vi "write_master_file.vi"(8 "error in (no error)":errorcluster, 10 "setup file paths":string, 11 "master file path":path) -> (0 "error out":errorcluster)   [LabVIEW 2017, in "worker.lvlib"]
uses:
  worker.lvlib
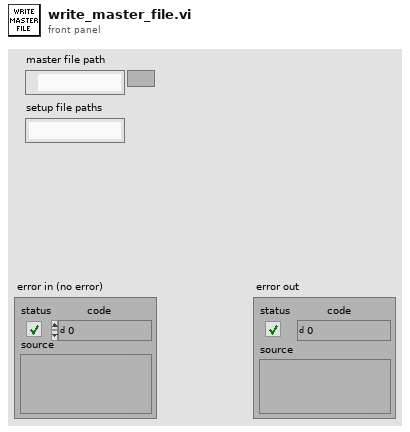
[diagram p1: front panel]
types:
  T1 = enum16{"open", "replace", "create", "open or create", "replace or create", "replace or create with confirmation"}
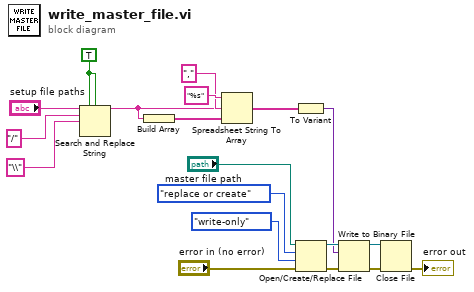
[diagram p0: block diagram]
diagram:
  w1 = TRUE ("replace all? (F)")
  n1 = Search and Replace String(replace all?=w1, case sensitive?=w1, input string="setup file paths", search string="/", replace string="\\" ("replace string (\"\")")) -> (result string=w4:string)  [unwired: 3 in, 3 out]
  n2 = Build Array(w4) -> (w8:string[])
  n3 = Spreadsheet String To Array(delimiter (Tab)=",", format string="%s", spreadsheet string=w4, array type (2D Dbl)=w8) -> (array=w6:string[])
  n4 = To Variant(anything=w6) -> (Variant=w13:variant)
  n5 = Open/Create/Replace File(file path (use dialog)="master file path", error in="error in (no error)", operation (0:open)=T1."replace or create", access (0:read/write)=enum16{"read/write", "read-only", "write-only"}."write-only") -> (refnum out=w14:refnum<file>, error out=w15:errorcluster)  [unwired: 2 in, 1 out]
  n6 = Write to Binary File(file (use dialog)=w14, data=w13, error in=w15) -> (refnum out=w11:refnum<file>, error out=w12:errorcluster)  [unwired: 3 in, 1 out]
  n7 = Close File(refnum=w11, error in=w12) -> (error out=→"error out":errorcluster)  [unwired: 1 out]
